vi "AprilTag Desktop.vi"() -> ()   [LabVIEW 2023]
uses:
  filter Selector.ctl
  <vilib>/Analysis/baseanly.llb/Real Inverse Matrix.vi
  <vilib>/Analysis/NI_AALBase.lvlib
  <vilib>/vision/driver/NI_Vision_Acquisition_Software.lvlib
panel:
  in  "Circles":bool
  in  "Chords":bool
  in  "Lines":bool
  in  "IMU offset":dbl
  out "Tags":T1(array[cluster])
  out "Field":cluster{cluster{"X":dbl, "Y":dbl}[]}[](graph)
  in  "Annotate":bool=TRUE
  in  "Hilite":bool=TRUE
  out "Camera IDs":string[](array[string])
  in  "Choose Camera":u16(ring) items=["FaceTime HD Camera (Built-in)  (#3E4BA11C5950E955).icd", "file::foo.png", "file::X3 back of stage with annotate.png", "file::X3 back of stage.png", "file::X3 back stage feed side.png", "file::X3 back stage.png", "file::X3 Calibration 1.png", "file::X3 calibration 2.png", "file::X3 midfield amp side.png", "file::X3 midfield feed side.png", "file::X3 midfield no annotate.png", "file::X3 protected stage point at feed no annotate.png", "file::X3 protected stage point at feed.png", "file::X3 stage.png", "file::X3 subwoofer no annotate.png", "file::X3 subwoofer.png"]
  in  "Hamming cutoff":i32
  in  "filter":T2
  out "Y (in)":dbl format="%.1f"
  out "Z (in)":dbl format="%.1f"
  out "X (in)":dbl format="%.1f"
  in  "Length (in)":dbl=100.0
  in  "width (in)":dbl=100.0
  out "Picture":picture
  in  "show rejects":bool
  out "bad":i32
  out "loop time (s)":dbl
  in  "Scale to Inches":dbl[](array[numeric])=[2.5, 2.5, 2.5]
  out "Chart of positional info":T3(graph)
  out "YPR (deg)":cluster{"yaw":dbl, "pitch":dbl, "roll":dbl} {"yaw" format="%.1f"; "pitch" format="%.1f"; "roll" format="%.1f"}
  out "ofsets (in)":cluster{"X":dbl, "Y":dbl, "Z":dbl} {"X" format="%.1f"; "Y" format="%.1f"; "Z" format="%.1f"}
  in  "Intrinsic Camera Matrix":dbl[][](array[numeric])=[[1135.0, 0.0, 640.0], [0.0, 1135.0, 360.0], [0.0, 0.0, 1.0]]
  out "good":i32
  in  "Tag Familys":string[](array[combo])=["16h5"]
  in  "blur":dbl step=0.1
  in  "refine Edges":bool=TRUE
  in  "decimate":dbl=4.0
  in  "threads":i32=2
  out "search time (s)":dbl
  out "good tag details":T4(array[cluster])
  in  "score cutoff":dbl(slide)=60.60606060606061 scale=0.0..100.0
  out "Image":T5(plugin-control)
  # "Angles between\ntarget and camera"
  # "Better way to pick camera matrix\ncheck other cams and simplify scaling"
  # "Offset between\ntarget and camera"
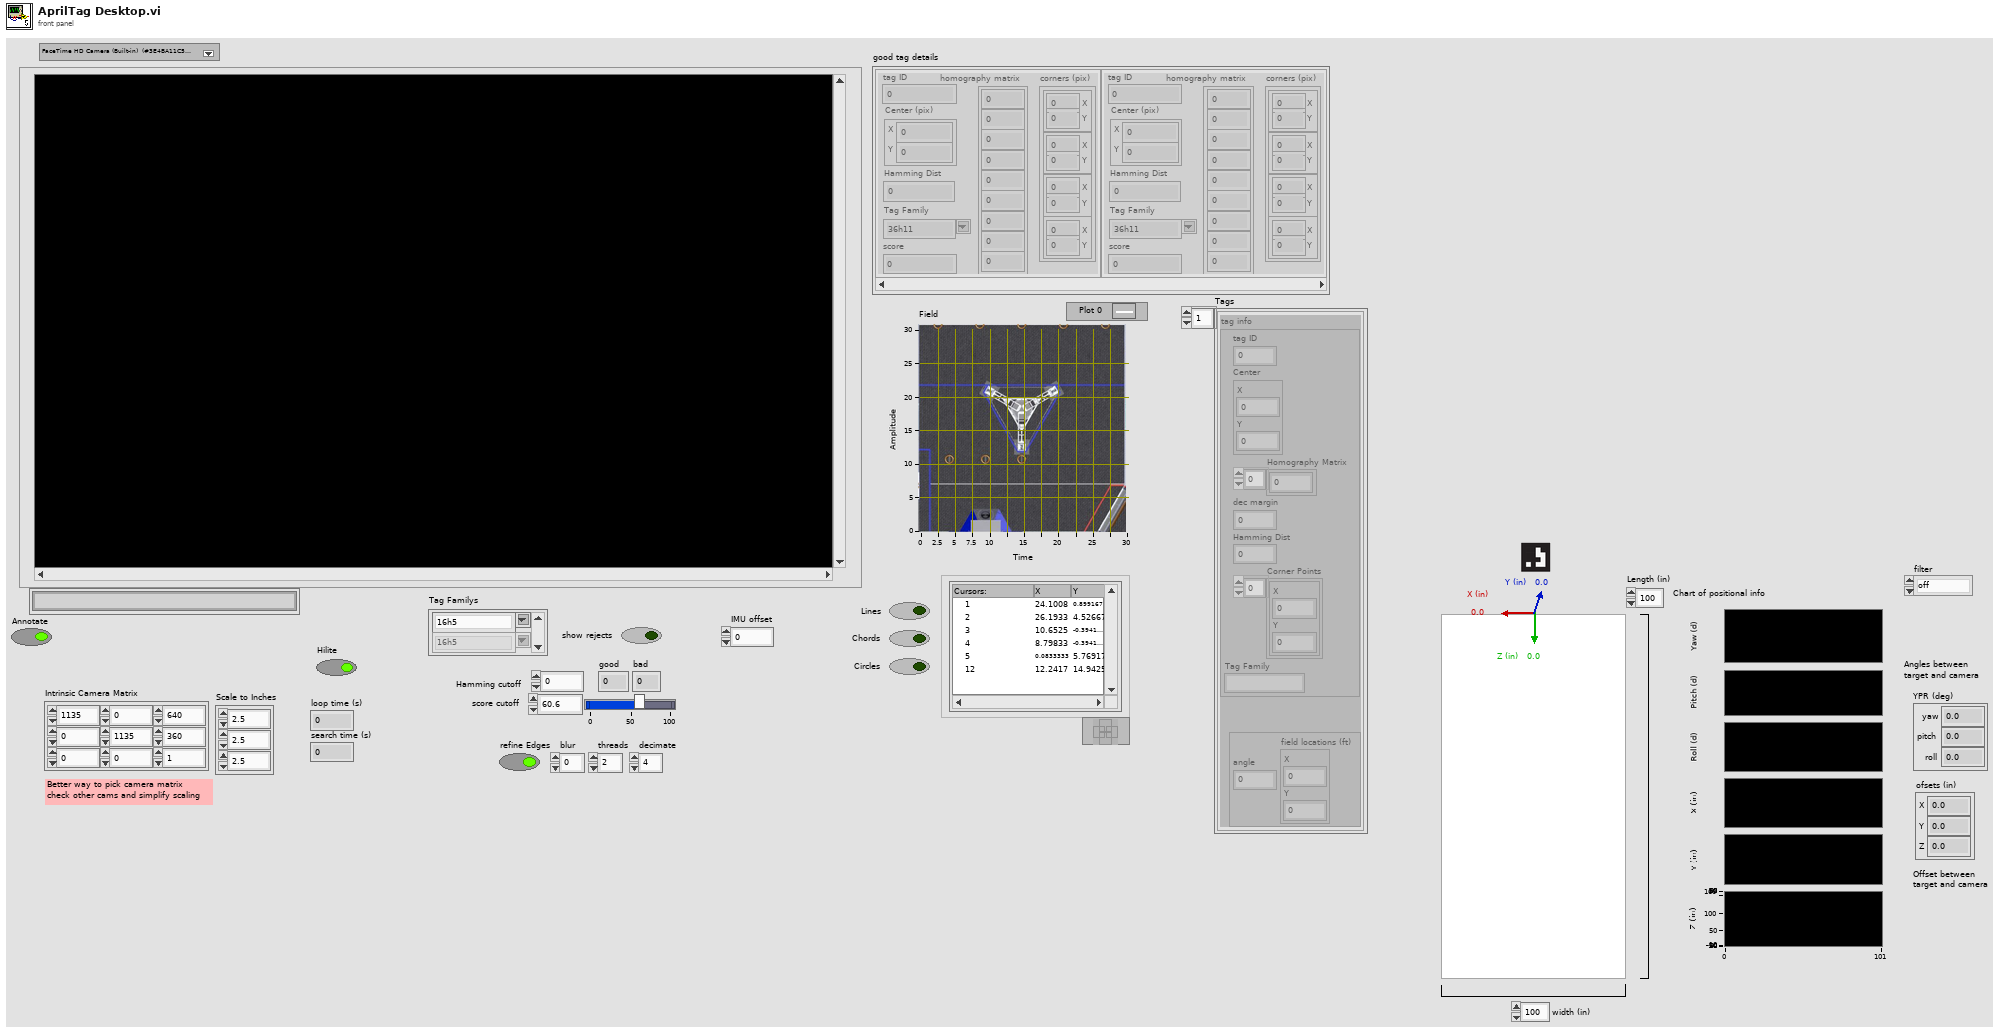
[diagram p1: front panel]
types:
  T1 = cluster{"tag info":cluster{"tag ID":i32, "Center":cluster{"X":dbl, "Y":dbl}, "Homography Matrix":dbl[], "dec margin":dbl, "Hamming Dist":i32, "Corner Points":cluster{"X":dbl, "Y":dbl}[], "Tag Family":string}, cluster{"angle":dbl, "field locations (ft)":cluster{"X":dbl, "Y":dbl}}}[]
  T2 = typedef "filter Selector.ctl" = enum16{"off", "2 pt avg", "low pass"}
  T3 = cluster{"yaw":dbl, "pitch":dbl, "roll":dbl, dbl, dbl, dbl}
  T4 = cluster{"tag ID":i32, "Center (pix)":cluster{"X":dbl, "Y":dbl}, "homography matrix":dbl[], "score":dbl, "Hamming Dist":i32, "corners (pix)":cluster{"X":dbl, "Y":dbl}[], "Tag Family":string}[]
  T5 = typedef "IMAQ Image.ctl" = refnum<image>
  T6 = cluster{i32, "Position":cluster{"X":dbl, "Y":dbl}}[]
  T7 = cluster{"Name":string, u32, "Style":i32, "Point Style":i32, "Name Visible":bool, "Allow Drag":bool, "Cursor Mode":u32, "Plot":i32, "Index":i32, "Position":cluster{"X":dbl, "Y":dbl}, "X Scale":u32, "Y Scale":u32, "Watch Plots":i32[], "Watch All Plots":bool, "Plot Area":i32, "Label Offset":cluster{"X":i32, "Y":i32}}
  T8 = cluster{"Type":u32, "Version":u32, "Flags":u32, "SerialNumberHigh":u32, "SerialNumberLow":u32, "BusType":u32, "InterfaceName":string, "VendorName":string, "ModelName":string, "CameraFileName":string, "CameraAttributeURL":string}[]
  T9 = typedef "Image Type" = u32
  T10 = cluster{"tag ID":i32, "Center":cluster{"X":dbl, "Y":dbl}, "homography matrix":dbl[], "decision margin":dbl, "Hamming Dist":i32, "corner points":cluster{"X":dbl, "Y":dbl}[], "Tag Family":string}[]
  T11 = cluster{"Hamming cutoff":i32, "score cutoff":dbl, "show rejects":bool}
  T12 = cluster{"tag ID":i32, "Center":cluster{"X":dbl, "Y":dbl}, "Homography Matrix":dbl[], "dec margin":dbl, "Hamming Dist":i32, "Corner Points":cluster{"X":dbl, "Y":dbl}[], "Tag Family":string}[]
  T13 = cluster{"tag info":cluster{"tag ID":i32, "Center":cluster{"X":dbl, "Y":dbl}, "Homography Matrix":dbl[], "dec margin":dbl, "Hamming Dist":i32, "Corner Points":cluster{"X":dbl, "Y":dbl}[], "Tag Family":string}, cluster{"angle":dbl, "field locations (ft)":cluster{"X":dbl, "Y":dbl}}}
  T14 = cluster{cluster{"tag info":cluster{"tag ID":i32, "Center":cluster{"X":dbl, "Y":dbl}, "Homography Matrix":dbl[], "dec margin":dbl, "Hamming Dist":i32, "Corner Points":cluster{"X":dbl, "Y":dbl}[], "Tag Family":string}, cluster{"angle":dbl, "field locations (ft)":cluster{"X":dbl, "Y":dbl}}}, cluster{"tag info":cluster{"tag ID":i32, "Center":cluster{"X":dbl, "Y":dbl}, "Homography Matrix":dbl[], "dec margin":dbl, "Hamming Dist":i32, "Corner Points":cluster{"X":dbl, "Y":dbl}[], "Tag Family":string}, cluster{"angle":dbl, "field locations (ft)":cluster{"X":dbl, "Y":dbl}}}}
  T15 = typedef "NI_Matrix.lvlib/RealMatrix.ctl" = dbl[][]
  T16 = typedef "LVBoundsTypeDef.ctl" = cluster{"Width":u32, "Height":u32}
  T17 = cluster{"tag ID":i32, "Center":cluster{"X":dbl, "Y":dbl}, "Homography Matrix":dbl[], "dec margin":dbl, "Hamming Dist":i32, "Corner Points":cluster{"X":dbl, "Y":dbl}[], "Tag Family":string}
  T18 = cluster{"Translation[0]":dbl, "Translation[1]":dbl, "Translation[2]":dbl}
  T19 = cluster{"picture out":picture, "offset":cluster{dbl, dbl}}
  T20 = cluster{"angle":dbl, "field locations (ft)":cluster{"X":dbl, "Y":dbl}}
  T21 = cluster{cluster{"angle":dbl, "field locations (ft)":cluster{"X":dbl, "Y":dbl}}, cluster{"angle":dbl, "field locations (ft)":cluster{"X":dbl, "Y":dbl}}}
  T22 = cluster{"center":cluster{"X":sgl, "Y":sgl}, "radius":sgl}
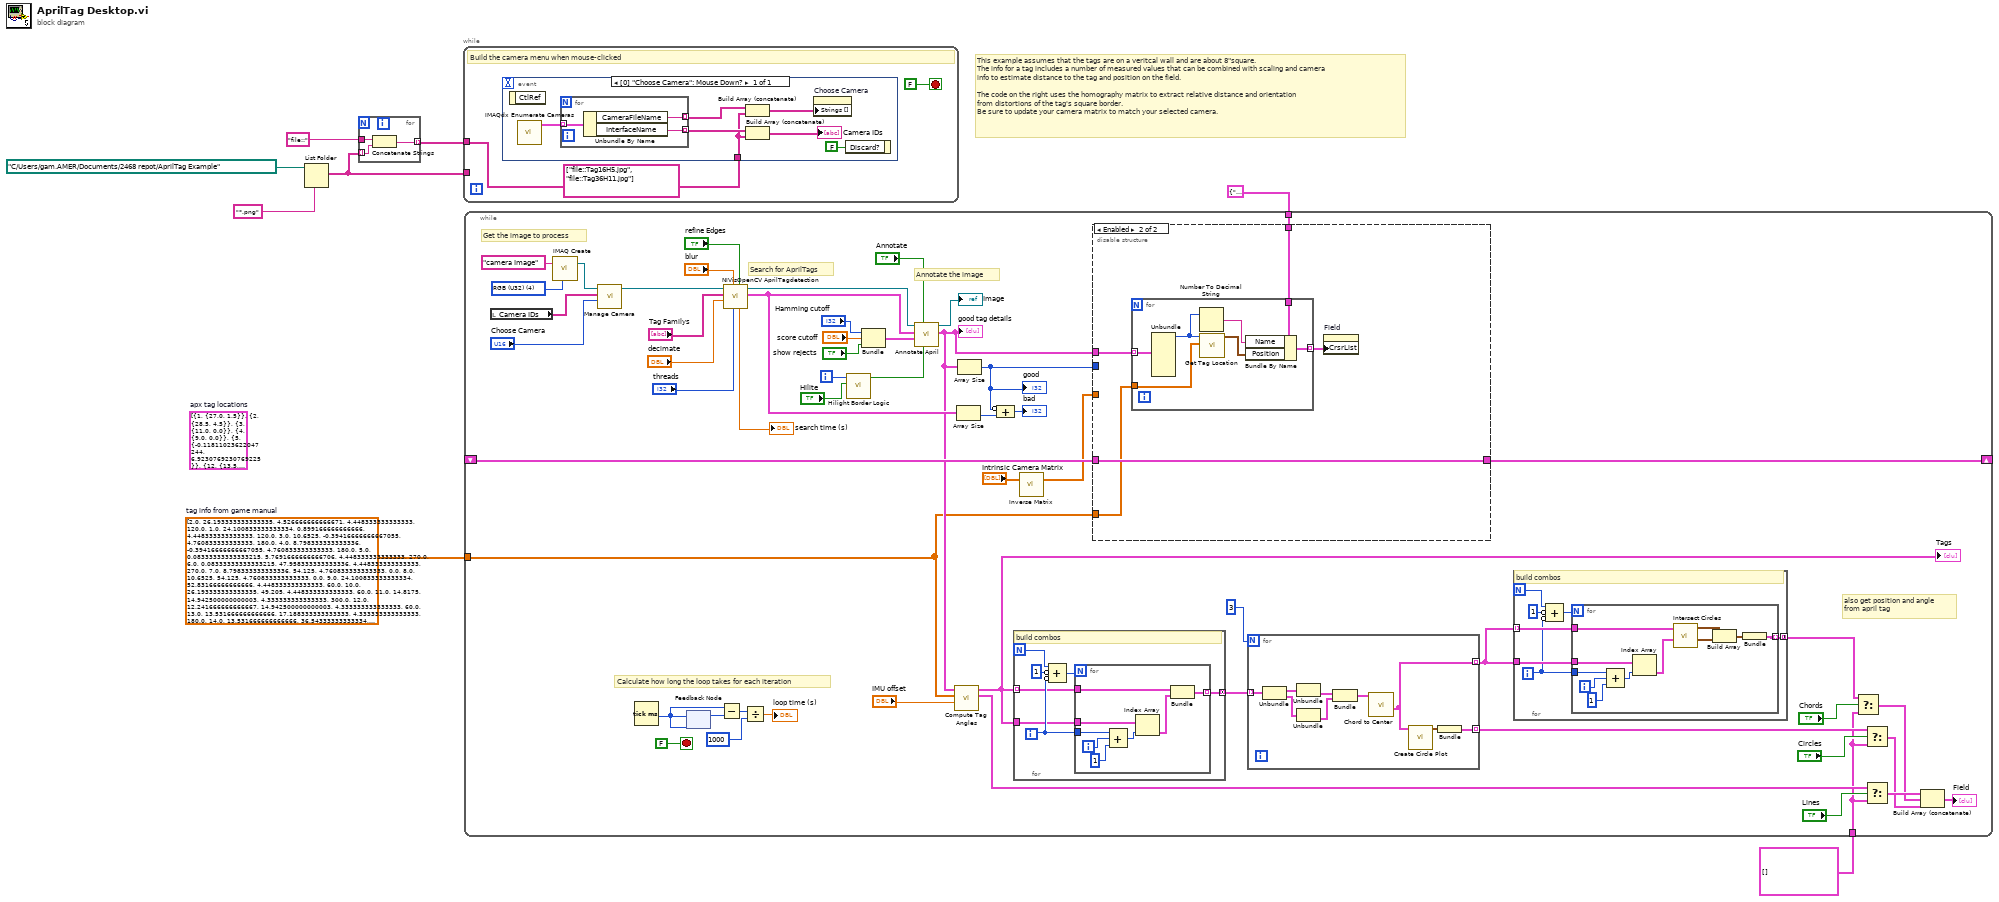
[diagram p0: block diagram]
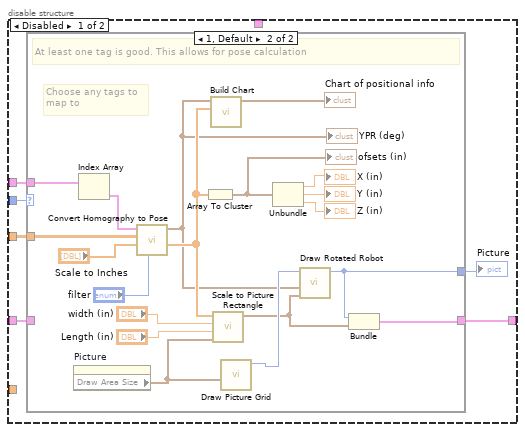
[diagram p2: hidden frame]
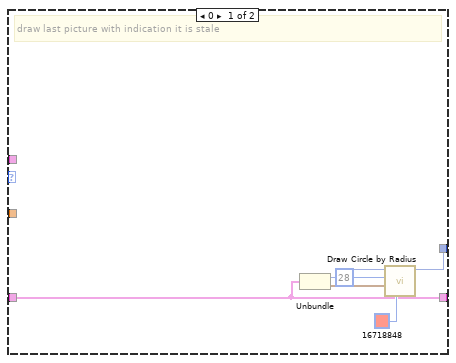
[diagram p3: hidden frame]
diagram:
  w1 = dbl[][] [[2.0, 26.193333333333335, 4.526666666666671, 4.448333333333333, 120.0], [1.0, 24.100833333333334, 0.899166666666666, 4.448333333333333, 120.0], [3.0, 10.6525, -0.39416666666667055, 4.760833333333333, 180.0], [4.0, 8.798333333333336, -0.39416666666667055, 4.760833333333333, 180.0], [5.0, 0.08333333333333215, 5.7691666666666706, 4.448333333333333, 270.0], [6.0, 0.08333333333333215, 47.958333333333336, 4.448333333333333, 270.0], [7.0, 8.798333333333336, 54.125, 4.760833333333333, 0.0], [8.0, 10.6525, 54.125, 4.760833333333333, 0.0], [9.0, 24.100833333333334, 52.83166666666666, 4.448333333333333, 60.0], [10.0, 26.193333333333335, 49.205, 4.448333333333333, 60.0], [11.0, 14.8175, 14.942500000000003, 4.333333333333333, 300.0], [12.0, 12.241666666666667, 14.942500000000003, 4.333333333333333, 60.0], [13.0, 13.531666666666666, 17.188333333333333, 4.333333333333333, 180.0], [14.0, 13.531666666666666, 36.54333333333334, 4.333333333333333, 0.0], [15.0, 12.241666666666667, 38.7725, 4.333333333333333, 120.0], [16.0, 14.8175, 38.7725, 4.333333333333333, 240.0]]  # tag info from game manual
  (unwired) T6 [{1, "Position"={"X"=27.0, "Y"=1.5}}, {2, "Position"={"X"=28.5, "Y"=4.5}}, {3, "Position"={"X"=11.0, "Y"=0.0}}, {4, "Position"={"X"=9.0, "Y"=0.0}}, {5, "Position"={"X"=-0.11811023622047244, "Y"=6.9230769230769225}}, {12, "Position"={"X"=13.5, "Y"=17.0}}]  # apx tag locations
  # "This example assumes that the tags are on a veritcal wall and are about 8\"square. \nThe info for a tag includes a number of measured values that can be combined with scaling and camera\ninfo to estimate distance to the tag and position on the field. \n\nThe code on the right uses the homography matrix to extract relative distance and orientation\nfrom distortions of the tag's square border.\nBe sure to update your camera matrix to match your selected camera."
  n1 = List Folder(path=path "C:/Users/gam.AMER/Documents/2468 repot/AprilTag Example", pattern="*.png") -> (filenames=w5:string[])  [unwired: 2 in, 3 out]
  n2 = for {
    tunnel: "file::" -> [w11]
    tunnel: w5 -> [w10] mode=indexing
    tunnel: [w9] -> w4 mode=indexing
    n3 = Concatenate Strings(w11, w10) -> (w9:string)
  }
  n4 = while {
    tunnel: w5 -> [_]
    tunnel: w4 -> [w12]
    stop <- FALSE stop-if-true
    (unwired) string[] ["file::Tag16H5.jpg", "file::Tag36H11.jpg"]
    # "Build the camera menu when mouse-clicked"
    n5 = event shown="[0] \"Choose Camera\": Mouse Down?" {
      selector: _ -> [_]
      dyn-events: _ -> [_]
      timeout: _ -> [_]
      tunnel: w12 -> [w15]
      event "Choose Camera": Mouse Down? {
        n6 = event-data() -> ()  [unwired: 1 in, 1 out]
        n7 = call <vilib>:"IMAQdx Enumerate Cameras.vi"() -> ("Camera Information Array"=w20:T8)  [unwired: 10 in, 1 out]
        n8 = for {
          tunnel: w20 -> [w23] mode=indexing
          tunnel: [w22] -> w19 mode=indexing
          tunnel: [w21] -> w17 mode=indexing
          n9 = Unbundle By Name(w23) -> ("CameraFileName"=w22:string, "InterfaceName"=w21:string)
        }
        n10 = Build Array (concatenate)(w19, w15) -> (w18:string[])
        n11 = Build Array (concatenate)(w17, w15) -> (→"Camera IDs":string[])
        n12 = property on="Choose Camera" class="Ring (strict)"("Strings []"=w18) -> ()  [unwired: 2 in, 2 out]
        n13 = event-data("Discard?"=FALSE) -> ()  [unwired: 1 in, 1 out]
      }
    }
  }
  n14 = while {
    shift-right: [w72] -> _
    shift-left: _ -> [w73]
    tunnel: T7 {"Name"="", 61192, "Style"=4, "Point Style"=6, "Name Visible"=TRUE, "Allow Drag"=TRUE, "Cursor Mode"=0, "Plot"=0, "Index"=0, "Position"={"X"=0.0, "Y"=0.0}, "X Scale"=0, "Y Scale"=0, "Watch Plots"=[], "Watch All Plots"=FALSE, "Plot Area"=0, "Label Offset"={"X"=1, "Y"=1}} -> [w41]
    tunnel: w1 -> [w40]
    tunnel: cluster{cluster{"X":dbl, "Y":dbl}[]}[] [] ("Vectors") -> [w27]
    i -> [w59]
    stop <- FALSE stop-if-true
    w46 = T9 4 items=["Grayscale (U8)", "Grayscale (I16)", "Grayscale (SGL)", "Complex (CSG)", "RGB (U32)", "HSL (U32)", "RGB (U64)", "Grayscale (U16)"] ("Image Type")
    # "also get position and angle\nfrom april tag"
    # "Calculate how long the loop takes for each iteration"
    # "Annotate the image"
    # "Search for AprilTags"
    # "Get the image to process"
    n15 = local read "Camera IDs"() -> (w52:string[])
    n16 = call "IMAQ Create"("Image Name"="camera Image", "Image Type"=w46) -> ("New Image"=w45:T5)  [unwired: 3 in, 1 out]
    n17 = call "Manage Camera.vi"("Choose Camera"="Choose Camera", "Camera IDs"=w52, "Image in"=w45) -> ("Image out"=w78:T5)  [unwired: 8 in]
    n18 = Tick Count (ms)() -> (millisecond timer value=w70:u32)
    n19 = feedback-in #1(w70) -> ()
    n20 = feedback #1(w70) -> (w71:u32)
    n21 = Subtract(x=w70, y=w71) -> (x-y=w62:u32)
    n22 = call <vilib>:"NIVisOpenCV AprilTagdetection.vi"("refine Edges"="refine Edges", "threads"="threads", "blur"="blur", "decimate"="decimate", "Tag Familys"="Tag Familys", "Image Src"=w78) -> ("Detected Tags"=w53:T10, "Image Dst Out"=w77:T5, "exec time (s)"=→"search time (s)":dbl)  [unwired: 2 in, 1 out]
    n23 = Divide(x=w62, y=1000) -> (x/y=→"loop time (s)":dbl)
    n24 = call "Hilight Border Logic.vi"("Hilight"="Hilite", "index"=w59) -> ("Hilight"=w58:bool)  [unwired: 9 in]
    n25 = Bundle("Hamming cutoff"="Hamming cutoff", "score cutoff"="score cutoff", "show rejects"="show rejects") -> (w54:T11)  [unwired: 1 in]
    n26 = call "Annotate April.vi"("hilight"=w58, "Annotate"="Annotate", "cutoffs"=w54, "Detected Tags"=w53, "Refnum in"=w77) -> ("tags"=w42:T12, "Refnum out"=→"Image":T5)  [unwired: 4 in, 1 out]
    "good tag details" <- w42
    n27 = call "Compute Tag Angles.vi"("IMU offset"="IMU offset", "tag info"=w40, "located tags"=w42) -> ("Vectors"=w35:cluster{cluster{"X":dbl, "Y":dbl}[]}[], "updated tags"=w37:T1)  [unwired: 7 in]
    "Tags" <- w37
    n28 = Array Size(array=w53) -> (size(s)=w69:i32)
    n29 = Array Size(array=w42) -> (size(s)=w50:i32)
    "good" <- w50
    n30 = Compound Arithmetic op=ADD(invert w50, w69) -> (→"bad":i32)
    n31 = for {
      N -> [w106]
      tunnel: [w112] -> w38 mode=concatenating
      tunnel: w37 -> [w108] mode=indexing
      tunnel: w37 -> [w107]
      i -> [w110]
      # "build combos"
      n32 = Compound Arithmetic op=ADD(w106, invert 1 ("value"), invert w110) -> (w111:i32)
      n33 = for {
        N: w111 -> [_]
        tunnel: w110 -> [w118]
        tunnel: [w115] -> w112 mode=indexing
        tunnel: w108 -> [w114]
        tunnel: w107 -> [w113]
        i -> [w117]
        n34 = Compound Arithmetic op=ADD(w118, w117, 1 ("value")) -> (w119:i32)
        n35 = Index Array(array=w113, index=w119) -> (element=w120:T13)
        n36 = Bundle(w114, w120) -> (w115:T14)  [unwired: 1 in]
      }
    }
    n37 = call-poly <vilib>:"Inverse Matrix.vi"("Input Matrix"="Intrinsic Camera Matrix") -> ("Inverse Matrix"=w48:T15)  [unwired: 1 in, 1 out]
    n38 = disable-structure shown="Enabled" {
      disable-tunnel: w73 -> [w125 w155]
      disable-tunnel: [w124 w155] -> w72
      disable-tunnel: w50 -> [w123 _]
      disable-tunnel: w48 -> [w122 _]
      disable-tunnel: w42 -> [w121 w156]
      disable-tunnel: w41 -> [_ w154]
      disable-tunnel: w40 -> [_ w152]
      frame Disabled {
        n39 = case shown="1, Default" w123 {
          tunnel: w122 -> [_ w151]
          tunnel: [w132 w147] -> w126
          tunnel: w125 -> [w127 _]
          tunnel: [w127 w146] -> w124
          tunnel: w121 -> [_ w145]
          frame 0 {
            # "draw last picture with indication it is stale"
            n40 = Unbundle(w127) -> ("picture out"=w131:picture, "offset"=w130:cluster{dbl, dbl})
            n41 = call <vilib>:"Draw Circle by Radius.vi"("color(black)"=u32 16718848, "pixel center"=w130, "radius"=i16 28, "picture"=w131) -> ("new picture"=w132:picture)  [unwired: 7 in]
          }
          frame 1, Default {
            # "Choose any tags to\nmap to"
            # "At least one tag is good. This allows for pose calculation"
            n42 = property on="Picture" class="Pict"() -> ("Draw Area Size"=w136:T16)  [unwired: 2 in, 2 out]
            n43 = Index Array(array=w145) -> (element=w135:T17)  [unwired: 1 in]
            n44 = call "Convert Homography to Pose.vi"("filter"="filter", "Scale to Inches"="Scale to Inches", "Inverse Camera Matrix"=w151, "tag info"=w135) -> ("Translation"=w137:dbl[], "angles (deg)"=w134:cluster{"yaw":dbl, "pitch":dbl, "roll":dbl})  [unwired: 5 in, 1 out]
            "YPR (deg)" <- w134
            n45 = Array To Cluster(array=w137) -> (cluster=w138:T18)
            "ofsets (in)" <- w138
            n46 = call "Build Chart.vi"("Translation"=w137, "angles (deg)"=w134) -> ("chart data"=→"Chart of positional info":T3)  [unwired: 9 in]
            n47 = call "Scale to Picture Rectangle.vi"("Draw Area Size"=w136, "Length (in)"="Length (in)", "width (in)"="width (in)", "Translation XYZ"=w137) -> ("offset"=w142:cluster{dbl, dbl})  [unwired: 7 in]
            n48 = call "Draw Picture Grid.vi"("Draw Area Size"=w136) -> ("picture out"=w144:picture)  [unwired: 10 in]
            n49 = Unbundle(w138) -> ("Translation[0]"=→"X (in)":dbl, "Translation[1]"=→"Y (in)":dbl, "Translation[2]"=→"Z (in)":dbl)
            n50 = call "Draw Rotated Robot.vi"("offset"=w142, "YPR (deg)"=w134, "Picture in"=w144) -> ("picture out"=w147:picture)  [unwired: 8 in]
            n51 = Bundle("picture out"=w147, "offset"=w142) -> (w146:T19)  [unwired: 1 in]
          }
        }
        "Picture" <- w126
      }
      frame Enabled {
        n52 = for {
          tunnel: w156 -> [w163] mode=indexing
          tunnel: w152 -> [w162]
          tunnel: w154 -> [w161]
          tunnel: [w159] -> w153 mode=indexing
          n53 = Unbundle(w163) -> ("tag ID"=w157:i32)  [unwired: 6 out]
          n54 = Number To Decimal String(number=w157) -> (decimal integer string=w158:string)  [unwired: 1 in]
          n55 = call "Get Tag Location.vi"("tag info"=w162, "tag ID"=w157) -> ("field locations (ft)"=w160:cluster{"X":dbl, "Y":dbl})  [unwired: 9 in]
          n56 = Bundle By Name(cluster=w161, "Name"=w158, "Position"=w160) -> (w159:T7)
        }
        n57 = property on="Field" class="XYGraph (strict)"("CrsrList"=w153) -> ()  [unwired: 2 in, 2 out]
      }
    }
    n58 = for {
      N: 3 -> [_]
      tunnel: w38 -> [w105] mode=indexing
      tunnel: [w99] -> w32 mode=indexing
      tunnel: [w97] -> w26 mode=indexing
      n59 = Unbundle(w105) -> (w104:T13, w103:T13)
      n60 = Unbundle(w104) -> (w98:T20)  [unwired: 1 out]
      n61 = Unbundle(w103) -> (w102:T20)  [unwired: 1 out]
      n62 = Bundle(w98, w102) -> (w101:T21)  [unwired: 1 in]
      n63 = call "Chord to Center.vi"("Tag points"=w101) -> ("output circle info"=w97:T22)  [unwired: 7 in, 3 out]
      n64 = call "Create Circle Plot.vi"("Circle Descr"=w97) -> ("Points"=w100:cluster{dbl, dbl}[])  [unwired: 10 in]
      n65 = Bundle("Points"=w100) -> (w99:cluster{"Points":cluster{dbl, dbl}[]})  [unwired: 1 in]
    }
    n66 = for {
      N -> [w80]
      tunnel: w26 -> [w85] mode=indexing
      tunnel: w26 -> [w84]
      tunnel: [w79] -> w25 mode=concatenating
      i -> [w82]
      # "build combos"
      n67 = Compound Arithmetic op=ADD(w80, invert 1 ("value"), invert w82) -> (w83:i32)
      n68 = for {
        N: w83 -> [_]
        tunnel: w85 -> [w91]
        tunnel: w84 -> [w96]
        tunnel: w82 -> [w94]
        tunnel: [w87] -> w79 mode=indexing
        i -> [w93]
        n69 = Compound Arithmetic op=ADD(w94, w93, 1 ("value")) -> (w95:i32)
        n70 = Index Array(array=w96, index=w95) -> (element=w90:T22)
        n71 = call "Intersect Circles.vi"("Circle 2"=w90, "Circle 1"=w91) -> ("Point 2"=w88:cluster{dbl, dbl}, "Point 1"=w89:cluster{dbl, dbl})  [unwired: 8 in]
        n72 = Build Array(w89, w88) -> (w86:cluster{dbl, dbl}[])
        n73 = Bundle(w86) -> (w87:cluster{cluster{dbl, dbl}[]})  [unwired: 1 in]
      }
    }
    n74 = Select(t=w25, s="Chords", f=w27) -> (s? t:f=w30:cluster{cluster{"X":dbl, "Y":dbl}[]}[])
    n75 = Select(t=w32, s="Circles", f=w27) -> (s? t:f=w31:cluster{"Points":cluster{"X":dbl, "Y":dbl}[]}[])
    n76 = Select(t=w35, s="Lines", f=w27) -> (s? t:f=w34:cluster{cluster{"X":dbl, "Y":dbl}[]}[])
    n77 = Build Array (concatenate)(w34, w30, w31) -> (→"Field":cluster{"Points":cluster{"X":dbl, "Y":dbl}[]}[])
  }
